vi "Use Filter Banks in Subband Coding.vi"() -> ()   [LabVIEW 2023]
doc: "This example demonstrates how to apply filter banks to subband coding applications. This example decomposes an audio signal into eight subband signals and allocates bits for each subband based on the variance.\n\nComplete the following steps to use this example:\n1) Specify the <b>Average Bits/Sample</b>.\n2) Run this VI.\n3) In the dialog box, select Sample1.wav and click the <b>OK</b> button to close the dialog box.\n4) Observe the <b>Allocated Bits/Sample</b>, <b>Variance</b>, and <b>Power Spectrum</b> of each subband. The higher the amplitude of <b>Variance</b> and <b>Power Spectrum</b>, the more bits are allocated.\n5) Run this VI. In the dialog box, select Sample2.wav.\n6) Observe the <b>Allocated Bits/Sample</b>, <b>Variance</b>, and <b>Power Spectrum</b> of each subband. Due to the higher variance, the fifth subband has more allocated bits."
uses:
  <vilib>/Analysis/4window.llb/windowTd.ctl
  <vilib>/sound2/lvsound2.llb/Sound File Info (path).vi
  <vilib>/measure/maspectr.llb/FFT Power Spectrum for 1 Chan.vi
  <vilib>/addons/Digital Filter Design/FilterBank.llb/Process/DFD M-Band Filter Bank Decomposition (Wfm).vi
  <vilib>/addons/Digital Filter Design/NI_DigFilter_FilterBank.lvlib
  <vilib>/measure/NI_MAPro.lvlib
  <vilib>/Analysis/NI_AALPro.lvlib
panel:
  out "Variance":dbl[](graph)
  in  "Average Bits/Sample":i32=5
  out "Power Spectrum":cluster{"f0":dbl, "df":dbl, "magnitude":dbl[]}(graph)
  out "Allocated Bits/Sample":dbl[](array[numeric])
  # "Select Help>>Show Context Help and move the cursor over the VI icon for more information."
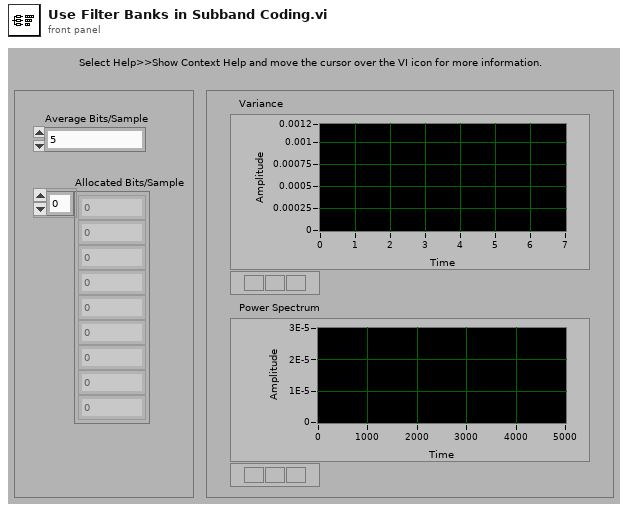
[diagram p1: front panel]
types:
  T1 = typedef "Sound Data Format.ctl" = cluster{"sample rate (S/s)":dbl, "number of channels":i32, "bits per sample":i32}
  T2 = typedef "NI_AALPro.lvlib/windowTd.ctl" = u32
  T3 = typedef "NI_DigFilter_FilterBank.lvlib/DFD Filter Bank Obj.ctl" = cluster{"mFBank_AnalysisFilters":T4[], "mFBank_SynthesisFilters":T4[], "mFBank_#Bands":i32, "mFBank_ProcMethod":T9, "mFBank_Coeffs":dbl[], "mFBank_Gain":dbl, "mFBank_Delay":i32, "mFBank_Type":T10}
  T4 = typedef "NI_DigFilterLicensed.lvlib/DFD Multirate Filter Obj.ctl" = cluster{"mMRate_Structure":enum16{"CIC", "FIR", "IIR", "Lattice"}, "mMRate_Mode":T5, "mMRate_Factor":i32, "mMRate_FIRParams":cluster{"mMRate_FIR_H":dbl[], "mMRate_FIR_IsNyquist?":bool, "mMRate_FIR_IsSymmetric?":bool}, "mMRate_CICParams":cluster{"mMRate_CIC_#Stage":i32, "mMRate_CIC_Lag":i32, "mMRate_CIC_Type":enum16{"Lowpass", "Highpass"}}, "mMRate_Order":i32, "mMRate_Version":string, "mMRate_Comments":string, "mMRate_RationalFactor":cluster{"mMRate_L":i32, "mMRate_M":i32}, "mMRate_Fs":dbl, "mMRate_Quantized?":bool, "mMRate_QFilterGain":dbl, "mMRate_CoefWl":i16, "mMRate_Scaling":cluster{"mMRate_ScaleByPowerOf2?":bool, "mMRate_ScaleType":T6}, "mMRate_InputWl":i16, "mMRate_OutputWl":i16, "mMRate_OutputMode":T7, "mMRate_MultMode":T8, "mMRate_BitPruning":bool, "mMRate_GainWl":i16, "mMRate_OutputFwl":i16, "mMRate_SumIwl":i16, "mMRate_InputIwl ":i16, "mMRate_SumWl":i16, "mMRate_CoefIwl":i16}
  T5 = typedef "NI_DigFilterLicensed.lvlib/DFD Multirate Mode.ctl" = i16
  T6 = typedef "NI_DigFilterLicensed.lvlib/DFD Coef Norm Type.ctl" = enum16{"No Norm", "Time Domain 1-Norm", "Time Domain 2-Norm", "Time Domain Inf-Norm"}
  T7 = typedef "NI_DigFilterLicensed.lvlib/DFD Round-off Mode.ctl" = enum16{"Nearest", "Truncation"}
  T8 = typedef "NI_DigFilterLicensed.lvlib/DFD FXP MRate Multiply Mode.ctl" = enum16{"Truncated", "Full"}
  T9 = typedef "NI_DigFilter_FilterBank.lvlib/DFD Filter Bank Processing Method.ctl" = enum16{"General", "2-Band QMF Lattice", "Cosine-Modulated"}
  T10 = typedef "NI_DigFilter_FilterBank.lvlib/DFD Filter Bank Type.ctl" = u16
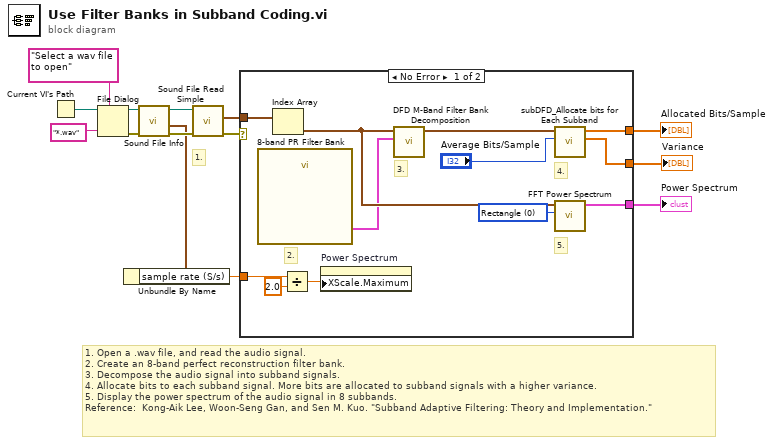
[diagram p0: block diagram]
diagram:
  # "1."
  # "1. Open a .wav file, and read the audio signal.\n2. Create an 8-band perfect reconstruction filter bank.\n3. Decompose the audio signal into subband signals.\n4. Allocate bits to each subband signal. More bits are allocated to subband signals with a higher variance. \n5. Display the power spectrum of the audio signal in 8 subbands.\nReference:  Kong-Aik Lee, Woon-Seng Gan, and Sen M. Kuo. \"Subband Adaptive Filtering: Theory and Implementation.\""
  n1 = Current VI's Path() -> (path=w14:path)
  n2 = File Dialog(6:"*.wav" ("pattern"), 7:"Select a wav file to open" ("prompt"), 11:w14) -> (0:w9:errorcluster, 3:w7:path)  [unwired: 1 in, 5 out]
  n3 = call-poly <vilib>:"Sound File Info.vi"("error in (no error)"=w9, "path"=w7) -> ("error out"=w8:errorcluster, "sound format"=w5:T1, "path out"=w6:path)  [unwired: 6 in, 1 out]
  n4 = Unbundle By Name(w5) -> ("sample rate (S/s)"=w4:dbl)
  n5 = call <vilib>:"Sound File Read Simple.vi"("error in (no error)"=w8, "path"=w6) -> ("error out"=w11:errorcluster, "data"=w10:waveform(dbl)[])  [unwired: 3 in, 5 out]
  n6 = case shown="No Error" w11 {
    tunnel: w10 -> [w18 _]
    tunnel: w4 -> [w24 _]
    tunnel: [w21 _] -> w2
    tunnel: [w20 _] -> w3
    tunnel: [w15 _] -> w1
    frame No Error {
      w26 = T2 0 items=["Rectangle"=0, "Hanning"=1, "Hamming"=2, "Blackman-Harris"=3, "Exact Blackman"=4, "Blackman"=5, "Flat Top"=6, "4 Term B-Harris "=7, "7 Term B-Harris"=8, "Low Sidelobe"=9, "Blackman Nuttall"=11, "Triangle"=30, "Bartlett-Hanning"=31, "Bohman"=32, "Parzen"=33, "Welch"=34, "Kaiser"=60, "Dolph-Chebyshev"=61, "Gaussian"=62] ("window")
      # "4."
      # "5."
      # "3."
      # "2."
      n7 = call "8-band PR Filter Bank"() -> ("filter bank out"=w19:T3)  [unwired: 10 in, 1 out]
      n8 = Index Array(array=w18) -> (element=w25:waveform(dbl))  [unwired: 1 in]
      n9 = Divide(x=w24, y=2.0) -> (x/y=w22:dbl)
      n10 = property on="Power Spectrum" class="WFGraph (strict)"("XScale.Maximum"=w22) -> ()  [unwired: 2 in, 2 out]
      n11 = call-poly <vilib>:"DFD M-Band Filter Bank Decomposition.vi"("filter bank in"=w19, "signal in"=w25) -> ("subband signals"=w17:waveform(dbl)[])  [unwired: 8 in, 1 out]
      n12 = call "subDFD_Allocate bits for Each Subband.vi"("average bits/sample"="Average Bits/Sample", "subband signals"=w17) -> ("variance"=w15:dbl[], "allocated bits/sample"=w21:dbl[])  [unwired: 8 in]
      n13 = call-poly <vilib>:"FFT Power Spectrum.vi"("window"=w26, "time signal"=w25) -> ("power spectrum"=w20:cluster{"f0":dbl, "df":dbl, "magnitude":dbl[]})  [unwired: 6 in, 3 out]
    }
    frame Error {
    }
  }
  "Power Spectrum" <- w3
  "Allocated Bits/Sample" <- w2
  "Variance" <- w1
